vi "oa_FIR Preprocess Filter Kaiser-Bessel Windowed FIR Filter De.vi"(7 "filter types":T2(ring), 8 "fs [Hz]":dbl=1.0, 10 "ripple specs [dB]":cluster{"pass band":dbl, "stop band":dbl}={"pass band"=0.1, "stop band"=60.0} {"stop band" format="%0.2f"; "pass band" format="%0.2f"}, 11 "freq specs [Hz]":T1={"fpass 1"=0.125, "fstop 1"=0.45, "fpass 2"=0.0, "fstop 2"=0.0} {"fstop 2" format="%0.2f"; "fpass 2" format="%.3f"; "fstop 1" format="%0.2f"; "fpass 1" format="%.3f"}) -> (0 "error":i32, 3 "FIR Windowed Coefficients":dbl[](array[numeric]) format="%0.2f")   [LabVIEW 2017, in "SoundVib_RefDataProcess.lvlib"]
uses:
  <vilib>/addons/Sound and Vibration/Order Analysis/Referece Data Processing/SoundVib_RefDataProcess.lvlib
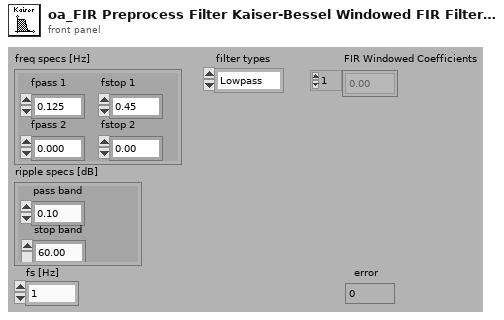
[diagram p1: front panel]
types:
  T1 = cluster{"fpass 1":dbl, "fstop 1":dbl, "fpass 2":dbl, "fstop 2":dbl}
  T2 = enum32{"Lowpass", "Highpass", "Bandpass", "Bandstop"}
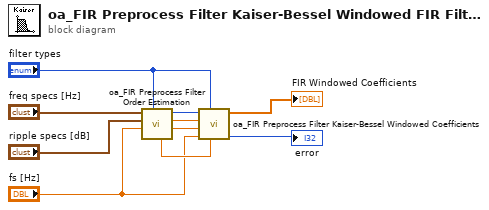
[diagram p0: block diagram]
diagram:
  n1 = call <vilib>:"oa_FIR Preprocess Filter Order Estimation.vi"("filter types"="filter types", "fs [Hz]"="fs [Hz]", "ripple specs [dB]"="ripple specs [dB]", "freq specs [Hz]"="freq specs [Hz]") -> ("low cutoff freq: fl"=w8:dbl, "high cutoff freq: fh"=w9:dbl, "estimated order"=w10:i32, "beta"=w7:dbl)  [unwired: 3 in, 1 out]
  n2 = call <vilib>:"oa_FIR Preprocess Filter Kaiser-Bessel Windowed Coefficients.vi"("beta"=w7, "filter type"="filter types", "sampling freq: fs"="fs [Hz]", "low cutoff freq: fl"=w8, "high cutoff freq: fh"=w9, "order"=w10) -> ("error"=→"error":i32, "FIR Windowed Coefficients"=→"FIR Windowed Coefficients":dbl[])  [unwired: 4 in]
